vi "RTM - Format Repeated Channel Alias.vi"(5 "AppendToChannels":bool, 7 "Instance":u32, 8 "error in (no error)":errorcluster, 10 "ChannelName":string, 11 "ExistingChannelNames":string[](array[string])=["lvc_current_command00", "lvc_current_command01", "lvc_current_command00_Instance01", "lvc_current_command01_Instance01"]) -> (0 "error out":errorcluster, 3 "FormattedName":string)   [LabVIEW 2019, in "UDP-Custom-Device System Explorer.lvlib"]
uses:
  UDP-Custom-Device System Explorer.lvlib
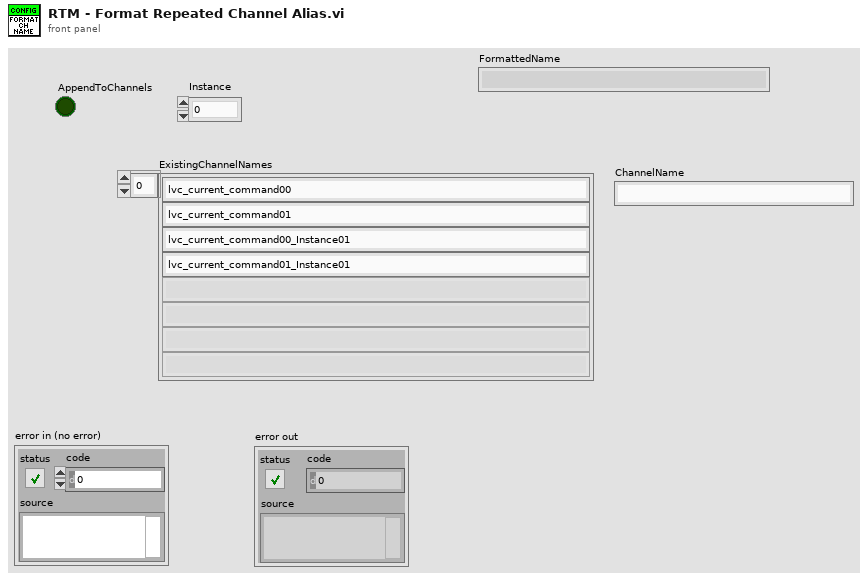
[diagram p1: front panel]
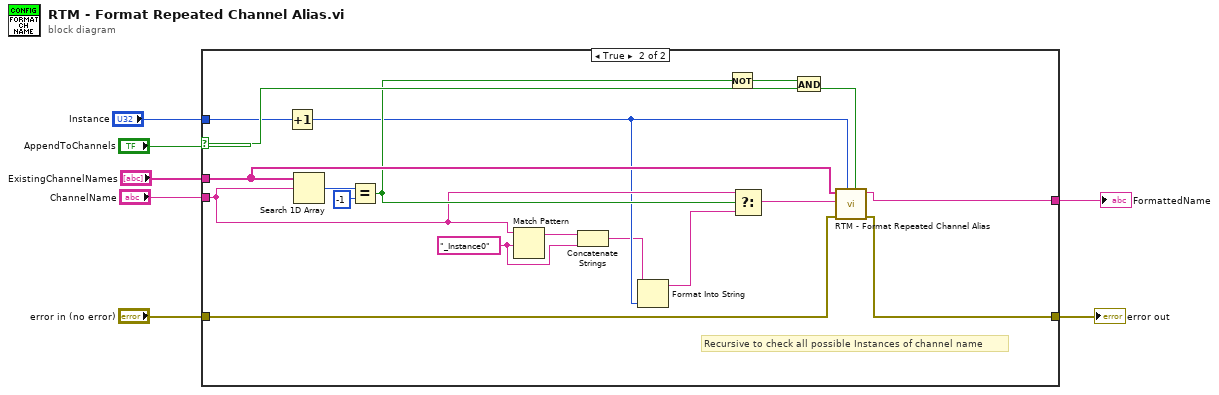
[diagram p0: block diagram]
diagram:
  n1 = case shown="True" "AppendToChannels" {
    selector: "AppendToChannels" -> [_ w24]
    tunnel: "error in (no error)" -> [w9 w15]
    tunnel: [w9 w14] -> w5
    tunnel: "ExistingChannelNames" -> [_ w23]
    tunnel: "ChannelName" -> [w8 w21]
    tunnel: "Instance" -> [_ w20]
    tunnel: [w8 w16] -> w1
    frame False {
    }
    frame True {
      w12 = "_Instance0" ("string")
      # "Recursive to check all possible Instances of channel name"
      n2 = Increment(x=w20) -> (x+1=w18:u32)
      n3 = Search 1D Array(1D array=w23, element=w21) -> (index of element=w27:i32)  [unwired: 1 in]
      n4 = Equal?(x=w27, y=-1) -> (x = y?=w22:bool)
      n5 = Match Pattern(string=w21, regular expression=w12) -> (before substring=w13:string)  [unwired: 1 in, 3 out]
      n6 = Concatenate Strings(w13, w12) -> (w11:string)
      n7 = Format Into String(initial string=w11, w18) -> (resulting string=w10:string)  [unwired: 2 in, 1 out]
      n8 = Not(x=w22) -> (.not. x?=w17:bool)
      n9 = Select(t=w21, s=w22, f=w10) -> (s? t:f=w25:string)
      n10 = And(x=w17, y=w24) -> (x .and. y?=w19:bool)
      n11 = call "RTM - Format Repeated Channel Alias.vi"("AppendToChannels"=w19, "Instance"=w18, "error in (no error)"=w15, "ChannelName"=w25, "ExistingChannelNames"=w23) -> ("error out"=w14:errorcluster, "FormattedName"=w16:string)  [unwired: 5 in]
    }
  }
  "error out" <- w5
  "FormattedName" <- w1
